vi "Arm Motor.vi"() -> ()   [LabVIEW 2010]
uses:
  <vilib>/NXT/Subs/MotorOutput.ctl
  <vilib>/NXT/Block Support/NXT_ButtonSelector.ctl
  <vilib>/NXT/Dual Mode Library/Motors/MotorBrake.vi
  <vilib>/NXT/Dual Mode Library/Sensors/readNXTButton.vi
  <vilib>/NXT/Dual Mode Library/Motors/MotorOn.vi
  <vilib>/NXT/Dual Mode Library/Sensors/Color_Detector.vi
  <vilib>/NXT/Dual Mode Library/Motors/Rotation.vi
panel:
  in  "stop":bool
  in  "Deg":i32
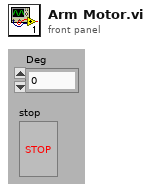
[diagram p1: front panel]
types:
  T1 = typedef "MotorOutput.ctl" = u8
  T2 = typedef "NXT_ButtonSelector.ctl" = u16
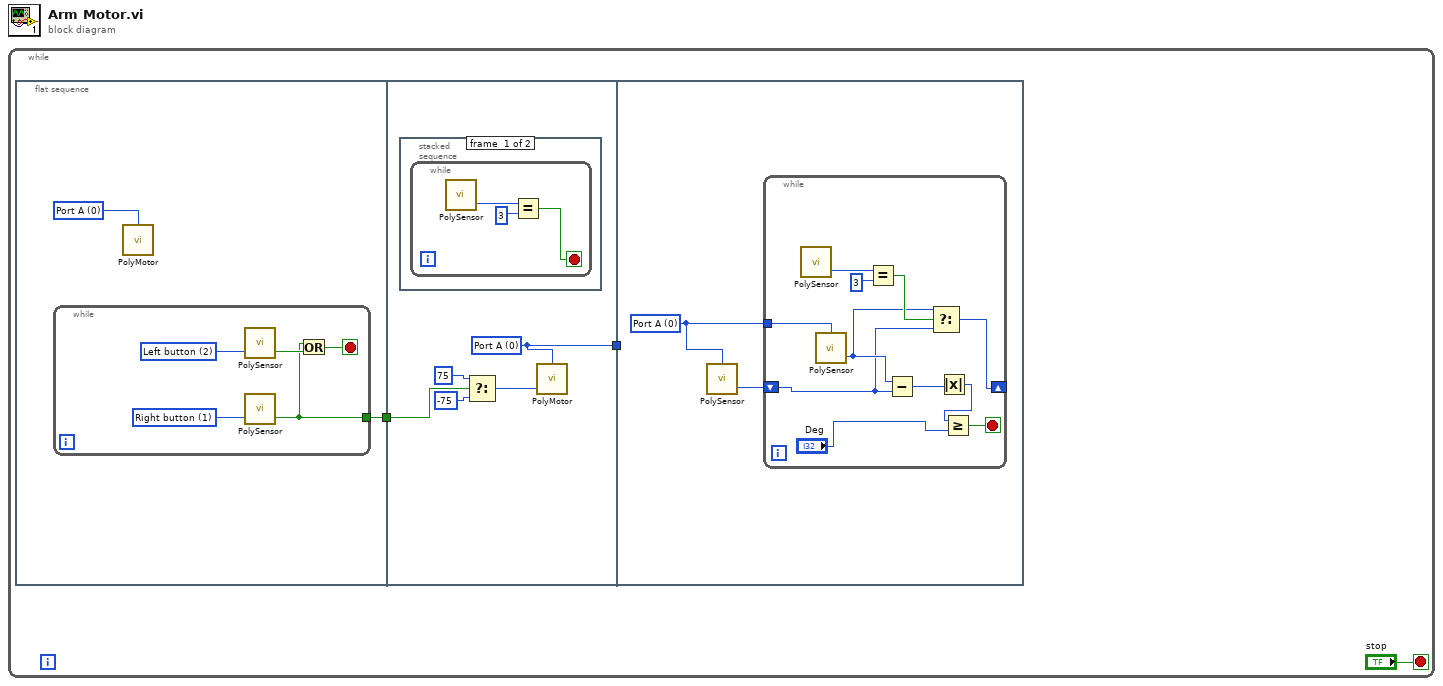
[diagram p0: block diagram]
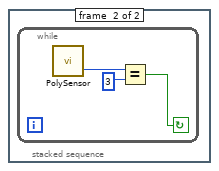
[diagram p2: hidden frame]
diagram:
  n1 = while {
    stop <- "stop" stop-if-true
    n2 = flat-sequence {
      tunnel: [w5] -> w3
      tunnel: w3 -> [w12]
      tunnel: [w11] -> w2
      tunnel: w2 -> [_]
      frame #0 {
        w4 = T1 0 items=["Port A"=0, "Port B"=1, "Port C"=2, "Ports A & B"=4, "Ports A & C"=5, "Ports B & C"=6, "All Ports"=3] ("Output Port (All Ports)")
        n3 = while {
          tunnel: [w6] -> w5
          stop <- w7 stop-if-true
          w9 = T2 1 items=["Enter button"=3, "Left button"=2, "Right button"=1] ("Button (Enter button)")
          w10 = T2 2 items=["Enter button"=3, "Left button"=2, "Right button"=1] ("Button (Enter button)")
          n4 = call-poly <vilib>:"PolySensor.vi"("Button (Enter button)"=w10) -> ("Yes/No"=w8:bool)  [unwired: 2 in, 1 out]
          n5 = call-poly <vilib>:"PolySensor.vi"("Button (Enter button)"=w9) -> ("Yes/No"=w6:bool)  [unwired: 2 in, 1 out]
          n6 = Or(x=w6, y=w8) -> (x .or. y?=w7:bool)
        }
        n7 = call-poly <vilib>:"PolyMotor.vi"("Port (All Ports)"=w4) -> ()  [unwired: 3 in, 1 out]
      }
      frame #1 {
        w11 = T1 0 items=["Port A"=0, "Port B"=1, "Port C"=2, "Ports A & B"=4, "Ports A & C"=5, "Ports B & C"=6, "All Ports"=3] ("Output Port (All Ports)")
        n8 = stacked-sequence {
          frame #0 {
            n9 = while {
              stop <- w16 stop-if-true
              n10 = call-poly <vilib>:"PolySensor.vi"() -> ("Detected Color"=w17:i16)  [unwired: 3 in, 1 out]
              n11 = Equal?(x=w17, y=i16 3) -> (x = y?=w16:bool)
            }
          }
          frame #1 {
            n12 = while {
              stop <- w19 continue-if-true
              n13 = call-poly <vilib>:"PolySensor.vi"() -> ("Detected Color"=w20:i16)  [unwired: 3 in, 1 out]
              n14 = Equal?(x=w20, y=i16 3) -> (x = y?=w19:bool)
            }
          }
        }
        n15 = Select(t=75, s=w12, f=-75 ("t")) -> (s? t:f=w15:i32)
        n16 = call-poly <vilib>:"PolyMotor.vi"("Power (75)"=w15, "Output Port (All Ports)"=w11) -> ()  [unwired: 2 in, 1 out]
      }
      frame #2 {
        w22 = u8 0 items=["Port A", "Port B", "Port C"] ("Port (Port A)")
        n17 = call-poly <vilib>:"PolySensor.vi"("Port (Port A)"=w22) -> ("Angle of Rotation"=w23:i32)  [unwired: 2 in, 1 out]
        n18 = while {
          tunnel: w22 -> [w33]
          shift-right: [w27] -> _
          shift-left: w23 -> [w24]
          stop <- w34 stop-if-true
          n19 = call-poly <vilib>:"PolySensor.vi"() -> ("Detected Color"=w28:i16)  [unwired: 3 in, 1 out]
          n20 = call-poly <vilib>:"PolySensor.vi"("Port (Port A)"=w33) -> ("Angle of Rotation"=w25:i32)  [unwired: 2 in, 1 out]
          n21 = Equal?(x=w28, y=i16 3) -> (x = y?=w26:bool)
          n22 = Subtract(x=w25, y=w24) -> (x-y=w32:i32)
          n23 = Select(t=w25, s=w26, f=w24) -> (s? t:f=w27:i32)
          n24 = Absolute Value(x=w32) -> (abs(x)=w31:i32)
          n25 = Greater Or Equal?(x=w31, y="Deg") -> (x >= y?=w34:bool)
        }
      }
    }
  }
